vi "transmit.vi"(8 "error in (no error)":errorcluster, 10 "Packets":string[](array[string]), 11 "UDP in":refnum<class "UDP Rx.lvclass">) -> (0 "error out":errorcluster, 3 "UDP out":refnum<class "UDP Rx.lvclass">)   [LabVIEW 2012, in "UDP Rx.lvclass"]
uses:
  UDP Rx.lvclass
  UDP Rx.lvclass/UDP Rx.ctl
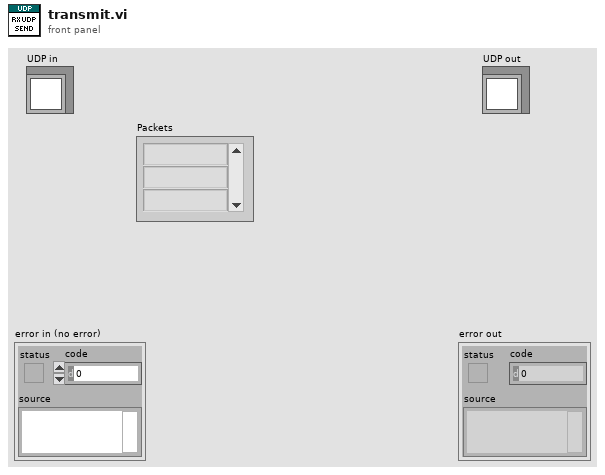
[diagram p1: front panel]
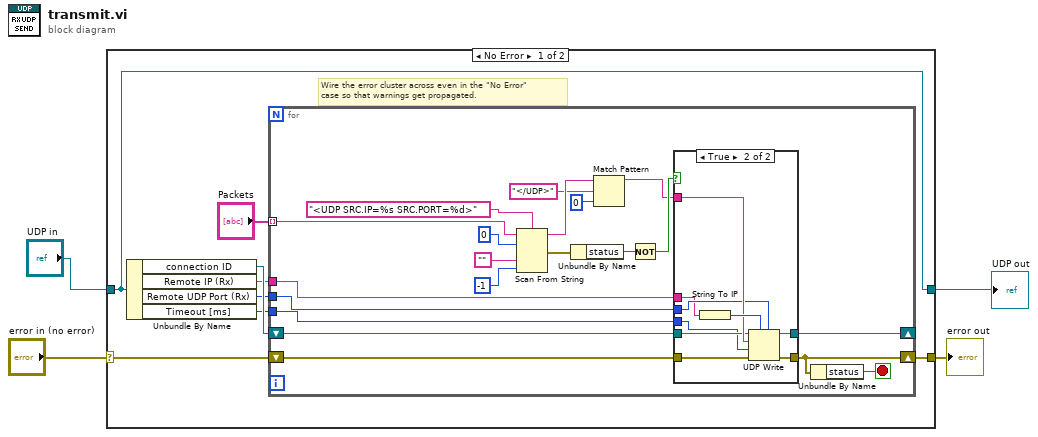
[diagram p0: block diagram]
diagram:
  n1 = case shown="No Error" "error in (no error)" {
    selector: "error in (no error)" -> [w12 w45]
    tunnel: [w11 w45] -> w3
    tunnel: [w10 w44] -> w1
    tunnel: "UDP in" -> [w10 w44]
    frame No Error {
      # "Wire the error cluster across even in the \"No Error\"\ncase so that warnings get propagated."
      n2 = Unbundle By Name(w10) -> ("connection ID"=w9:refnum<k16>, "Remote IP (Rx)"=w7:string, "Remote UDP Port (Rx)"=w8:u16, "Timeout [ms]"=w5:u16)
      n3 = for {
        shift-right: [w13] -> w11
        shift-left: w12 -> [w30]
        shift-right: [w32] -> _
        shift-left: w9 -> [w31]
        tunnel: w8 -> [w18]
        tunnel: w7 -> [w17]
        tunnel: "Packets" -> [w16] mode=indexing
        tunnel: w5 -> [w15]
        stop <- w14 stop-if-true
        n4 = Scan From String(format string="<UDP SRC.IP=%s SRC.PORT=%d>", input string=w16, initial scan location=u32 0, default 1="", default 2=-1 ("default value 2")) -> (remaining string=w22:string, error out=w25:errorcluster)  [unwired: 3 in, 1 out]
        n5 = Unbundle By Name(w25) -> ("status"=w28:bool)
        n6 = Match Pattern(string=w22, regular expression="</UDP>", offset (0)=0) -> (before substring=w19:string)  [unwired: 3 out]
        n7 = Not(x=w28) -> (.not. x?=w29:bool)
        n8 = case shown="True" w29 {
          tunnel: w19 -> [_ w42]
          tunnel: w31 -> [w34 w41]
          tunnel: [w34 w40] -> w32
          tunnel: [w33 w39] -> w13
          tunnel: w30 -> [w33 w38]
          tunnel: w18 -> [_ w37]
          tunnel: w17 -> [_ w36]
          tunnel: w15 -> [_ w35]
          frame False {
          }
          frame True {
            n9 = String To IP(1:w36) -> (0:w43:u32)
            n10 = UDP Write(address=w43, port or service name=w37, connection ID=w41, data in=w42, 8:w38, 9:w35) -> (error out=w39:errorcluster, 3:w40:refnum<k16>)
          }
        }
        n11 = Unbundle By Name(w13) -> ("status"=w14:bool)
      }
    }
    frame Error {
    }
  }
  "error out" <- w3
  "UDP out" <- w1
